vi "Script_NamesIOConstant.vi"() -> ()   [LabVIEW 2013]
panel:
  in  "ACTION":bool
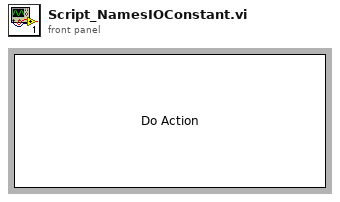
[diagram p1: front panel]
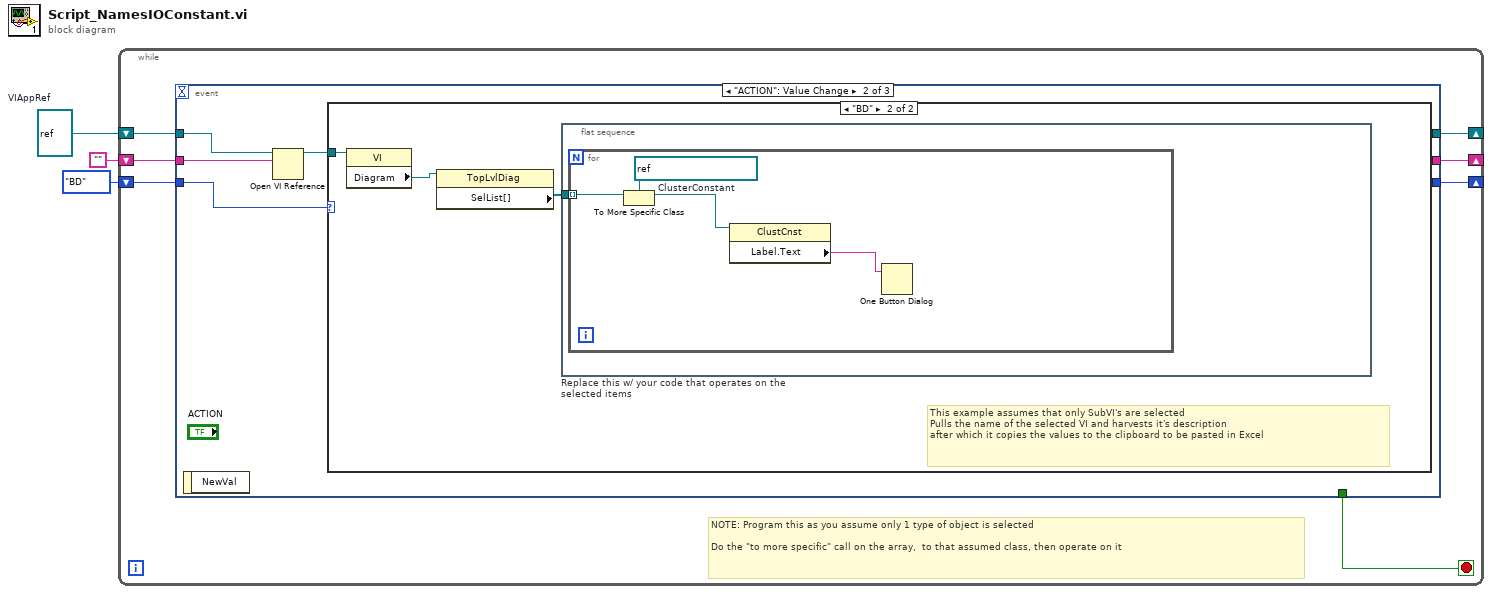
[diagram p0: block diagram]
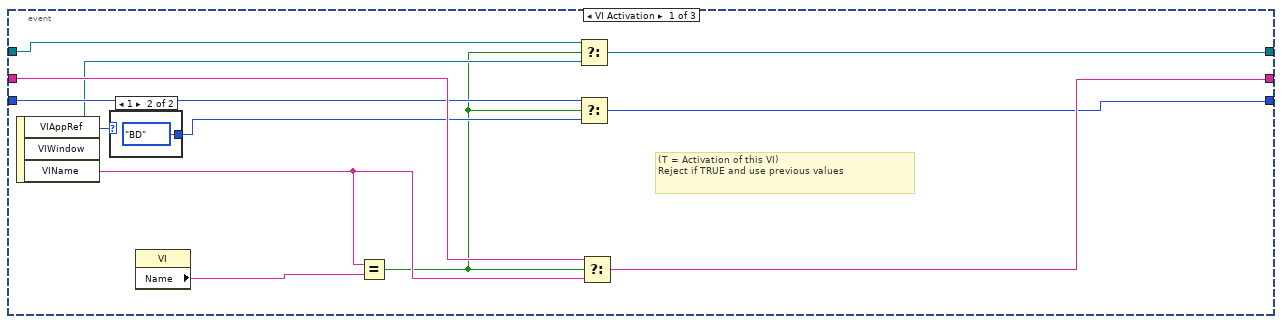
[diagram p2: hidden frame]
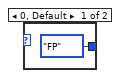
[diagram p3: hidden frame]
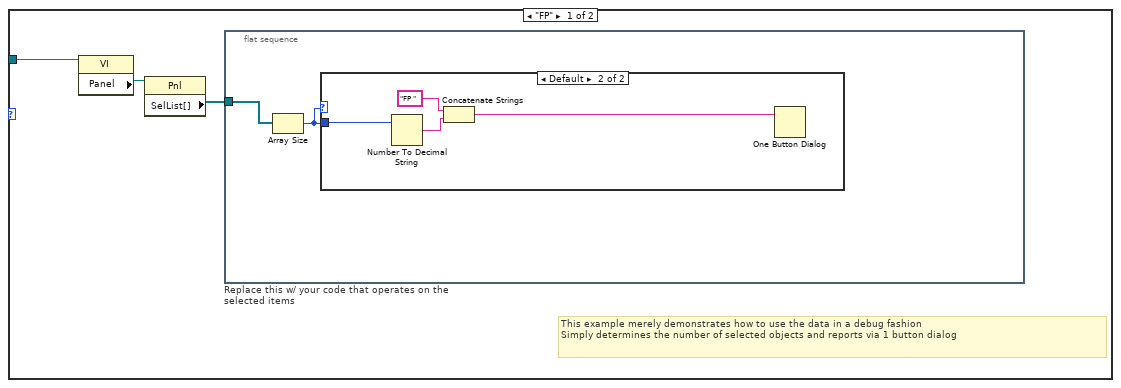
[diagram p4: hidden frame]
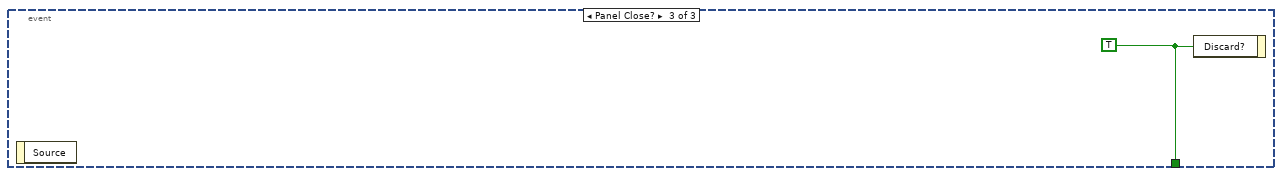
[diagram p6: hidden frame]
diagram:
  w1 = refnum<vi> refnum  # VIAppRef
  n1 = while {
    shift-right: [w10] -> _
    shift-left: "" -> [w9]
    shift-right: [w7] -> _
    shift-left: enum16{"FP", "BD"}."BD" -> [w6]
    shift-right: [w5] -> _
    shift-left: w1 -> [w4]
    stop <- w8 stop-if-true
    # "NOTE: Program this as you assume only 1 type of object is selected\n\nDo the \"to more specific\" call on the array,  to that assumed class, then operate on it"
    n2 = event shown="[1] \"ACTION\": Value Change" {
      selector: _ -> [_ _ _]
      dyn-events: _ -> [_ _ _]
      timeout: _ -> [_ _ _]
      tunnel: [w19 _ _] -> w10
      tunnel: w9 -> [w22 w28 _]
      tunnel: [_ _ w46] -> w8
      tunnel: [w17 _ _] -> w7
      tunnel: w6 -> [w18 w26 _]
      tunnel: [w13 _ _] -> w5
      tunnel: w4 -> [w12 w25 _]
      event VI Activation {
        # "(T = Activation of this VI)\nReject if TRUE and use previous values"
        n3 = event-data() -> ("VIAppRef"=w14:refnum<vi>, "VIWindow"=w16:i32, "VIName"=w20:string)  [unwired: 1 out]
        n4 = case shown="1" w16 {
          tunnel: [enum16{"FP", "BD"}."FP" enum16{"FP", "BD"}."BD"] -> w15
          frame 0, Default {
          }
          frame 1 {
          }
        }
        n5 = property class="VI"() -> ("Name"=w21:string)  [unwired: 2 in, 2 out]
        n6 = Equal?(x=w20, y=w21) -> (x = y?=w11:bool)
        n7 = Select(t=w12, s=w11, f=w14) -> (s? t:f=w13:refnum<vi>)
        n8 = Select(t=w18, s=w11, f=w15) -> (s? t:f=w17:enum16{"FP", "BD"})
        n9 = Select(t=w22, s=w11, f=w20) -> (s? t:f=w19:string)
      }
      event "ACTION": Value Change {
        n10 = event-data() -> ()  [unwired: 2 out]
        n11 = Open VI Reference(application reference (local)=w25, vi path=w28) -> (vi reference=w27:refnum<vi>)  [unwired: 2 in, 3 out]
        n12 = case shown="\"BD\"" w26 {
          tunnel: w27 -> [w31 w40]
          frame "FP" {
            # "This example merely demonstrates how to use the data in a debug fashion\nSimply determines the number of selected objects and reports via 1 button dialog"
            n13 = property class="VI"(reference=w31) -> ("Panel"=w30:refnum<vi>)  [unwired: 1 in, 2 out]
            n14 = property class="Pnl"(reference=w30) -> ("SelList[]"=w29:refnum<vi>[])  [unwired: 1 in, 2 out]
            n15 = flat-sequence "Replace this w/ your code that operates on the selected items" {
              tunnel: w29 -> [w32]
              frame #0 {
                n16 = Array Size(array=w32) -> (size(s)=w33:i32)
                n17 = case shown="Default" w33 {
                  tunnel: w33 -> [_ w37]
                  frame 0 {
                  }
                  frame Default {
                    n18 = Number To Decimal String(number=w37) -> (decimal integer string=w36:string)  [unwired: 1 out]
                    n19 = Concatenate Strings("FP " ("string"), w36) -> (w35:string)
                    n20 = One Button Dialog(message=w35) -> ()  [unwired: 2 out]
                  }
                }
              }
            }
          }
          frame "BD" {
            # "This example assumes that only SubVI's are selected\nPulls the name of the selected VI and harvests it's description\nafter which it copies the values to the clipboard to be pasted in Excel"
            n21 = property class="VI"(reference=w40) -> ("Diagram"=w39:refnum<vi>)  [unwired: 1 in, 2 out]
            n22 = property class="TopLvlDiag"(reference=w39) -> ("SelList[]"=w38:refnum<vi>[])  [unwired: 1 in, 2 out]
            n23 = flat-sequence "Replace this w/ your code that operates on the selected items" {
              tunnel: w38 -> [w41]
              frame #0 {
                n24 = for {
                  tunnel: w41 -> [w45] mode=indexing
                  w44 = refnum<vi> refnum  # ClusterConstant
                  n25 = To More Specific Class(target class=w44, reference=w45) -> (specific class reference=w43:refnum<vi>)  [unwired: 1 in, 1 out]
                  n26 = property class="ClustCnst"(reference=w43) -> ("Label.Text"=w42:string)  [unwired: 1 in, 2 out]
                  n27 = One Button Dialog(message=w42) -> ()  [unwired: 1 in, 1 out]
                }
              }
            }
          }
        }
      }
      event Panel Close? {
        w46 = TRUE ("Discard?")
        n28 = event-data() -> ()  [unwired: 2 out]
        n29 = event-data("Discard?"=w46) -> ()  [unwired: 1 in, 1 out]
      }
    }
  }
